vi "Base.vi"() -> ()   [LabVIEW 2022 SP3]
uses:
  Global 1 Base.vi
panel:
  out "Square":dynamicdata(graph)
  in  "stop (F)":bool
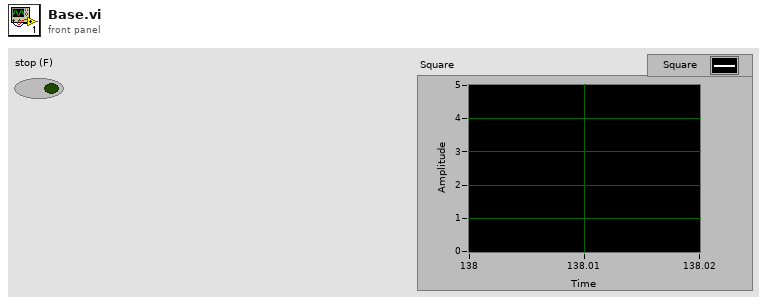
[diagram p1: front panel]
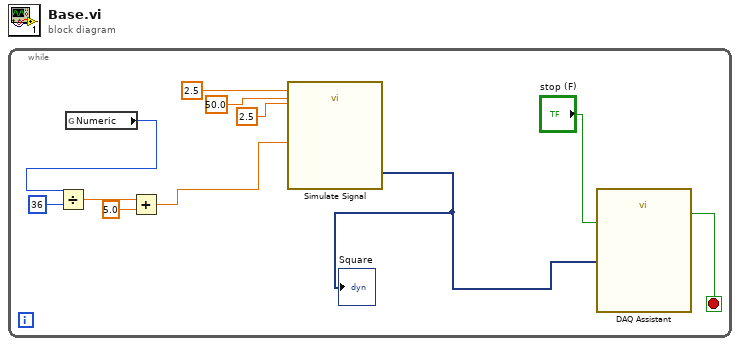
[diagram p0: block diagram]
diagram:
  n1 = while {
    stop <- w10 stop-if-true
    n2 = global read "Global 1 Base.vi" "Numeric"() -> (w1:i32)
    n3 = Divide(x=w1, y=36) -> (x/y=w2:dbl)
    n4 = Add(x=w2, y=5.0) -> (x+y=w3:dbl)
    n5 = call "Simulate Signal"("Offset"=2.5, "Duty Cycle (%)"=w3, "Frequency"=50.0, "Amplitude"=2.5) -> ("Square"=w9:dynamicdata)  [unwired: 10 in, 1 out]
    "Square" <- w9
    n6 = call "DAQ Assistant"("data"=w9, "stop (F)"="stop (F)") -> ("stopped"=w10:bool)  [unwired: 15 in, 2 out]
  }
